vi "Manual Shooter.vi"(10 "Joystick Refnum Name":string="My Joystick RefNum") -> ()   [LabVIEW 2016]
uses:
  <vilib>/Rock Robotics/WPI/Utilities/WPI_GetSetVariantRefNum.vi
  Robot Global Data.vi
panel:
  in  "D":dbl
  in  "I":dbl
  in  "P":dbl
  out "x/y":dbl
  in  "RPM":dbl
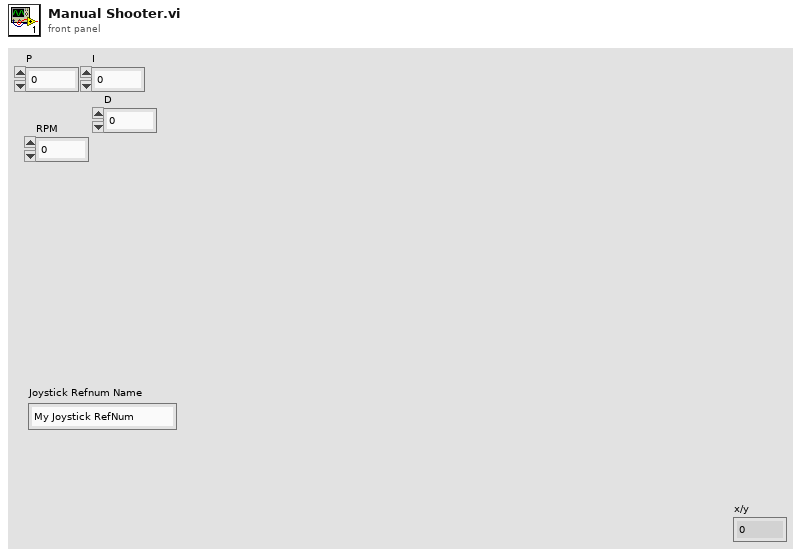
[diagram p1: front panel]
types:
  T1 = typedef "WPI_JoystickDevRef.ctl" = cluster{"Device":T2}
  T2 = typedef "WPI_JoystickDeviceEnum.ctl" = enum16{"USB 0", "USB 1", "USB 2", "USB 3", "USB 4", "USB 5"}
  T3 = typedef "WPI_MotorControlDeviceRef.ctl" = cluster{"DeviceStatus":errorcluster, "Type":T4, "PWM":cluster{"PWM Channel":T5, "DeadBand":T6}, "CAN":cluster{"Device Number":u8, "SetOutput VI Ref":variant, "GetOutput VI Ref":variant, "Enable VI Ref":variant, "Disable VI Ref":variant, "Data":variant}, "Invert":bool}
  T4 = typedef "WPI_MotorControlType.ctl" = enum16{"PWM", "CAN"}
  T5 = typedef "FPGA_DIOPWMChannel.ctl" = enum8{"PWM 0", "PWM 1", "PWM 2", "PWM 3", "PWM 4", "PWM 5", "PWM 6", "PWM 7", "PWM 8", "PWM 9", "PWM MXP 0", "PWM MXP 1", "PWM MXP 2", "PWM MXP 3", "PWM MXP 4", "PWM MXP 5", "PWM MXP 6", "PWM MXP 7", "PWM MXP 8", "PWM MXP 9", "Invalid"}
  T6 = typedef "WPI_PWMDeadband.ctl" = cluster{"Name":string, "maxPositivePwm":i32, "minPositivePwm":i32, "centerPwm":i32, "maxNegativePwm":i32, "minNegativePwm":i32, "angularRange":u16}
  T7 = typedef "WPI_CANTalonSRX_GlobalStatus.ctl" = cluster{"Applied Throttle":dbl, "Module Enabled":bool, "CAN Error":errorcluster, "Closed Loop Error":dbl, "Forward Limit Switch Closed":bool, "Reverse Limit Switch Closed":bool, "Sensor Position":dbl, "Sensor Velocity":dbl, "Current":dbl, "Sticky Fault - Over Temp":bool, "Sticky Fault - Under Voltage":bool, "Sticky Fault - Forward Limit":bool, "Sticky Fault - Reverse Limit":bool, "Sticky Fault - Forward Soft Limit":bool, "Sticky Fault - Reverse Soft Limit":bool, "Brake is Enabled":bool, "Encoder Position":dbl, "Encoder Velocity":dbl, "Encoder Index Count":dbl, "Encoder A Pin State":bool, "Encoder B Pin State":bool, "Encoder Index Pin State":bool, "Analog In":dbl, "Analog In Velocity":dbl, "Temperature (C)":dbl, "Battery Voltage":dbl, "Control 5 Is Supported":bool, "Current Profile Slot Select":dbl, "Pos Div 8":bool, "Vel Div 4":bool, "Pulse Width Position":i32, "Pulse Width Velocity":i32, "Pulse Width Rise To Rise (us)":i32, "Pulse Width Rise To Fall (us)":i32, "Mot Prof Active Is Under Run":bool, "Mot Prof Active Has Under Run":bool, "Mot Prof Active Is Last":bool, "Mot Prof Active Velocity Only":bool, "Mot Prof Active Is Valid":bool, "Mot Prof Buffer Is Full":bool, "Mot Prof Active Profile Slot Select":i32, "Mot Prof NextID":i32, "Mot Prof Count":i32, "Mot Prof Active Velocity":dbl, "Mot Prof Active Position":dbl, "Mot Prof Output Enable":i32}
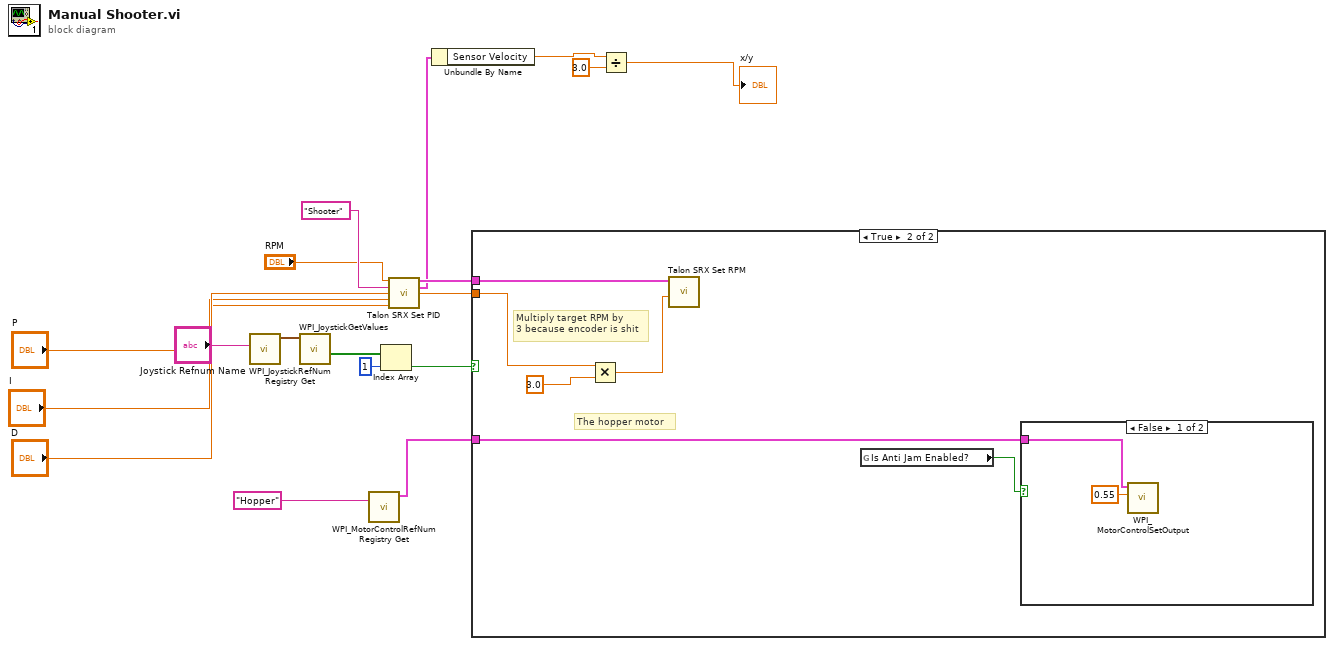
[diagram p0: block diagram]
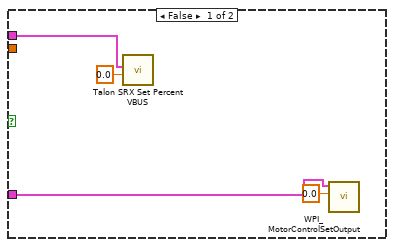
[diagram p2: hidden frame]
diagram:
  n1 = call <vilib>:"WPI_JoystickRefNum Registry Get.vi"("refnum name"="Joystick Refnum Name") -> ("JoystickDevRef"=w12:T1)  [unwired: 1 in, 9 out]
  n2 = call <vilib>:"WPI_JoystickGetValues.vi"("JoystickDevRef"=w12) -> ("Buttons"=w15:bool[])  [unwired: 6 in, 4 out]
  n3 = call <vilib>:"WPI_MotorControlRefNum Registry Get.vi"("refnum name"="Hopper") -> ("MotorControlDevRef"=w4:T3)  [unwired: 9 in, 1 out]
  n4 = Index Array(array=w15, index=1) -> (element=w14:bool)
  n5 = call "Talon SRX Set PID.vi"("Target RPM"="RPM", "Talon SRX Refnum Name"="Shooter", "P"="P", "I"="I", "D"="D") -> ("CAN Talon SRX Ref"=w17:T3, "Talon SRX Status"=w11:T7, "Target RPM Output"=w6:dbl)  [unwired: 7 in, 1 out]
  n6 = Unbundle By Name(w11) -> ("Sensor Velocity"=w9:dbl)
  n7 = case shown="True" w14 {
    tunnel: w17 -> [w22 w27]
    tunnel: w6 -> [_ w25]
    tunnel: w4 -> [w19 w23]
    frame False {
      n8 = call "Talon SRX Set Percent VBUS.vi"("Desired VBus"=0.0, "CAN Talon SRX Ref"=w22) -> ()  [unwired: 10 in]
      n9 = call <vilib>:"WPI_MotorControlSetOutput.vi"("Output"=0.0, "MotorControlDevRef"=w19) -> ()  [unwired: 7 in, 3 out]
    }
    frame True {
      # "The hopper motor"
      # "Multiply target RPM by \n3 because encoder is shit"
      n10 = Multiply(x=w25, y=3.0) -> (x*y=w26:dbl)
      n11 = call "Talon SRX Set RPM.vi"("Desired RPM"=w26, "CAN Talon SRX Ref"=w27) -> ()  [unwired: 10 in]
      n12 = global read "Robot Global Data.vi" "Is Anti Jam Enabled?"() -> (w24:bool)
      n13 = case shown="False" w24 {
        tunnel: w23 -> [w29 _]
        frame False {
          n14 = call <vilib>:"WPI_MotorControlSetOutput.vi"("Output"=0.55, "MotorControlDevRef"=w29) -> ()  [unwired: 7 in, 3 out]
        }
        frame True {
        }
      }
    }
  }
  n15 = Divide(x=w9, y=3.0) -> (x/y=→"x/y":dbl)
